vi "getReferenceFromName.vi"(8 "error in (no error)":errorcluster, 9 "referenceName":T1(ring), 10 "Pane":refnum<vi>, 11 "ICSettingsViewer in":refnum<class "ICSettingsViewer.lvclass">) -> (0 "error out":errorcluster, 1 "Ctl Refnum":refnum<vi>, 2 "Pane out":refnum<vi>, 3 "ICSettingsViewer out":refnum<class "ICSettingsViewer.lvclass">, 4 "found":bool)   [LabVIEW 2011, in "Views.lvlib" / "Camera.lvlib" / "ICSettingsViewer.lvclass"]
uses:
  ICSettingsViewer.lvclass
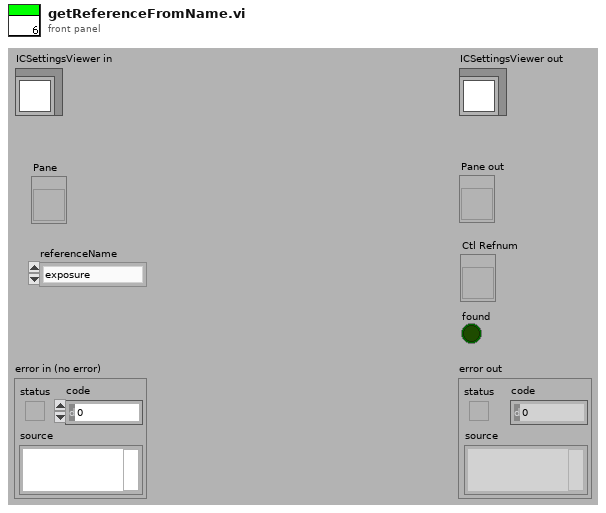
[diagram p1: front panel]
types:
  T1 = enum16{"exposure", "gain", "image_number", "Triggering", "start_trigger"}
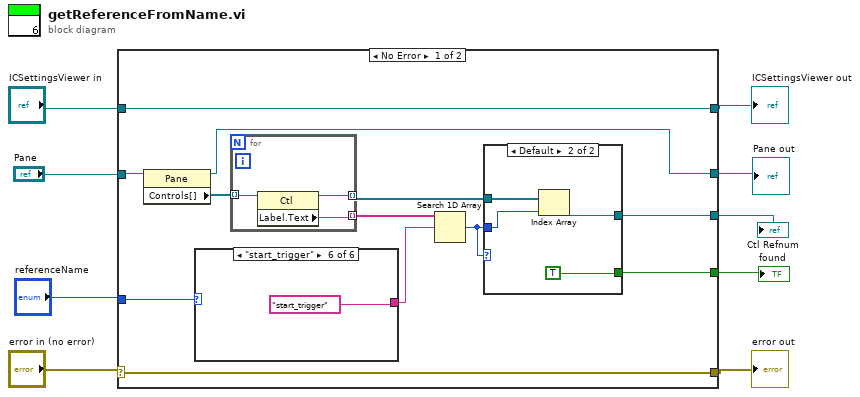
[diagram p0: block diagram]
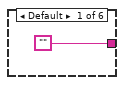
[diagram p2: hidden frame]
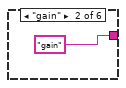
[diagram p3: hidden frame]
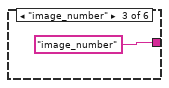
[diagram p4: hidden frame]
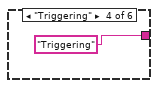
[diagram p5: hidden frame]
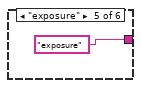
[diagram p6: hidden frame]
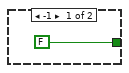
[diagram p7: hidden frame]
diagram:
  n1 = case shown="No Error" "error in (no error)" {
    selector: "error in (no error)" -> [w20 w37]
    tunnel: [w20 w37] -> w7
    tunnel: [w21 w36] -> w8
    tunnel: "ICSettingsViewer in" -> [w21 w36]
    tunnel: "Pane" -> [w19 _]
    tunnel: [w14 _] -> w3
    tunnel: [w13 _] -> w2
    tunnel: [w12 _] -> w5
    tunnel: "referenceName" -> [w11 _]
    frame No Error {
      n2 = property class="Pane"(reference=w19) -> (reference out=w12:refnum<vi>, "Controls[]"=w18:refnum<vi>[])  [unwired: 1 in, 1 out]
      n3 = case shown="\"start_trigger\"" w11 {
        tunnel: ["" "gain" "image_number" "Triggering" "exposure" "start_trigger"] -> w10
        frame Default {
        }
        frame "gain" {
        }
        frame "image_number" {
        }
        frame "Triggering" {
        }
        frame "exposure" {
        }
        frame "start_trigger" {
        }
      }
      n4 = for {
        tunnel: w18 -> [w35] mode=indexing
        tunnel: [w34] -> w17 mode=indexing
        tunnel: [w33] -> w16 mode=indexing
        n5 = property class="Ctl"(reference=w35) -> (reference out=w33:refnum<vi>, "Label.Text"=w34:string)  [unwired: 1 in, 1 out]
      }
      n6 = Search 1D Array(1D array=w17, element=w10) -> (index of element=w15:i32)  [unwired: 1 in]
      n7 = case shown="Default" w15 {
        tunnel: w16 -> [_ w32]
        tunnel: w15 -> [_ w31]
        tunnel: [FALSE TRUE] -> w14
        tunnel: [_ w29] -> w13
        frame -1 {
        }
        frame Default {
          n8 = Index Array(array=w32, index=w31) -> (element=w29:refnum<vi>)
        }
      }
    }
    frame Error {
    }
  }
  "error out" <- w7
  "ICSettingsViewer out" <- w8
  "Pane out" <- w5
  "found" <- w3
  "Ctl Refnum" <- w2
